vi "SetAttributeByName.vi"(8 "error in (no error)":errorcluster, 9 "Attribute":refnum<class "Attribute.lvclass">, 10 "AttrName":string, 11 "SMO in":refnum<class "SMO.lvclass">) -> (0 "error out":errorcluster, 1 "replaced":bool, 3 "SMO out":refnum<class "SMO.lvclass">)   [LabVIEW 2013, in "SMO.lvclass"]
uses:
  SMO.lvclass
  Support/Attribute/Attribute.lvclass
  Support/Attribute/Attribute.lvclass/Attribute.ctl
  <vilib>/Utility/LVClass/Get LV Class Name.vi
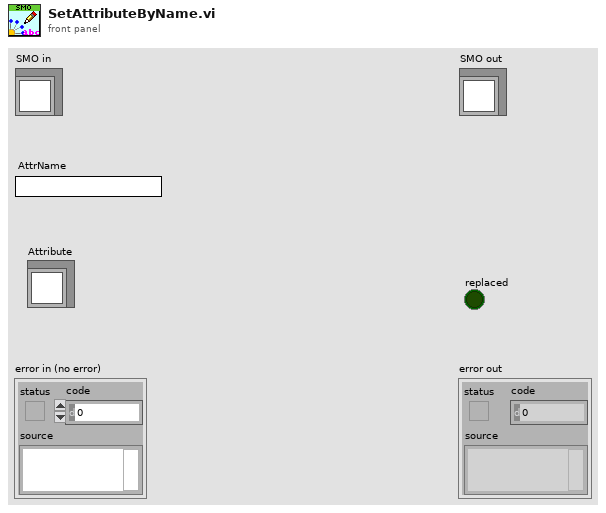
[diagram p1: front panel]
types:
  T1 = typedef "def.SMO.lvclass/Scope -- Enum.ctl" = enum16{"Public", "Protected", "Private"}
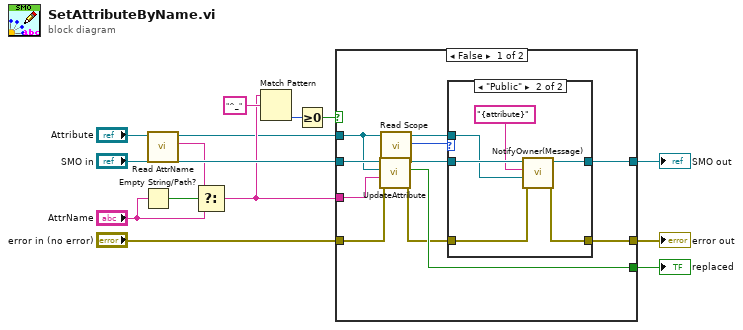
[diagram p0: block diagram]
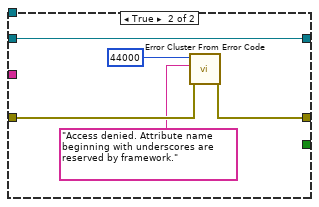
[diagram p3: hidden frame]
diagram:
  n1 = Empty String/Path?(string/path="AttrName") -> (empty?=w6:bool)
  n2 = call "Read AttrName.vi"("Attribute in"="Attribute") -> ("Attribute Name"=w1:string, "Attribute out"=w3:refnum<class "Attribute.lvclass">)  [unwired: 8 in, 1 out]
  n3 = Select(t=w1, s=w6, f="AttrName") -> (s? t:f=w5:string)
  n4 = Match Pattern(string=w5, regular expression="^_") -> (offset past match=w13:i32)  [unwired: 1 in, 3 out]
  n5 = Greater Or Equal To 0?(x=w13) -> (x >= 0?=w12:bool)
  n6 = case shown="False" w12 {
    tunnel: "error in (no error)" -> [w23 w37]
    tunnel: [w19 w38] -> w9
    tunnel: w5 -> [w24 _]
    tunnel: w3 -> [w18 _]
    tunnel: [w22 _] -> w11
    tunnel: "SMO in" -> [w25 w34]
    tunnel: [w20 w34] -> w10
    frame False {
      n7 = call "UpdateAttribute.vi"("error in (no error)"=w23, "Attribute Name"=w24, "Attribute"=w18, "SMO in"=w25) -> ("error out"=w15:errorcluster, "replaced"=w22:bool, "SMO out"=w21:refnum<class "SMO.lvclass">)  [unwired: 5 in]
      n8 = call "Read Scope.vi"("Attribute in"=w18) -> ("Scope"=w16:T1, "Attribute out"=w17:refnum<class "Attribute.lvclass">)  [unwired: 9 in]
      n9 = case shown="\"Public\"" w16 {
        tunnel: w21 -> [w27 w33]
        tunnel: [w27 w32] -> w20
        tunnel: w15 -> [w26 w28]
        tunnel: [w26 w29] -> w19
        tunnel: w17 -> [_ w30]
        frame Default {
        }
        frame "Public" {
          n10 = call "NotifyOwner(Message).vi"("error in (no error)"=w28, "Payload"=w30, "Message (empty : payload label)"="{attribute}" ("regular expression"), "SMO in"=w33) -> ("error out"=w29:errorcluster, "SMO out"=w32:refnum<class "SMO.lvclass">)  [unwired: 6 in]
        }
      }
    }
    frame True {
      n11 = call <vilib>:"Error Cluster From Error Code.vi"("error in (no error)"=w37, "error message (\"\")"="Access denied. Attribute name beginning with underscores are reserved by framework." ("error message (\"\")"), "error code (0)"=44000) -> ("error out"=w38:errorcluster)  [unwired: 6 in]
    }
  }
  "error out" <- w9
  "SMO out" <- w10
  "replaced" <- w11
